vi "PH_Powermeter_BaseClass.ProcEvents.vi"(0 "i ref in":refnum<vi>, 5 "error in":errorcluster) -> (14 "i ref out":refnum<vi>, 19 "error out":errorcluster)   [LabVIEW 2014, in "PH_Powermeter_BaseClass.lvlib"]
doc: "This method is used to define the events the object will listen to. Add your own events here."
uses:
  PH_Powermeter_BaseClass.lvlib
  CSCore/BaseProcess/BaseProcess.event definition.ctl
  CSCore/CAEObj/CAEObj.event definition.ctl
  CSCore/BaseProcess/BaseProcess.descriptor string definition.ctl
  CSCore/BaseProcess/BaseProcess.lvlib
  CSCore/CAEObj/CAEObj.lvlib
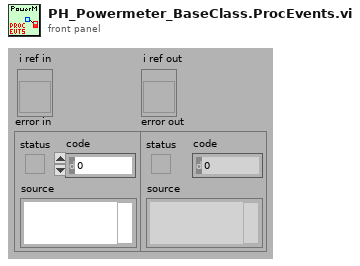
[diagram p1: front panel]
types:
  T1 = typedef "BaseProcess.lvlib/BaseProcess.event definition.ctl" = cluster{"CAEEvtDef":T2, "Data Descriptor":T3}
  T2 = typedef "CAEObj.lvlib/CAEObj.event definition.ctl" = cluster{"URL":string, "enable":bool, "ignoreResID":bool}
  T3 = typedef "BaseProcess.lvlib/BaseProcess.descriptor string definition.ctl" = string
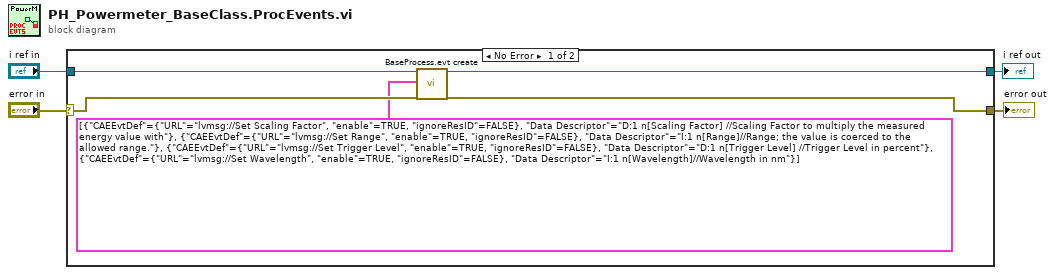
[diagram p0: block diagram]
diagram:
  n1 = case shown="No Error" "error in" {
    selector: "error in" -> [w7 w10]
    tunnel: "i ref in" -> [w6 w11]
    tunnel: [w9 w11] -> w3
    tunnel: [w8 w10] -> w2
    frame No Error {
      n2 = call "BaseProcess.evt create.vi"("i ref in"=w6, "newEvents"=T1[] [{"CAEEvtDef"={"URL"="lvmsg://Set Scaling Factor", "enable"=TRUE, "ignoreResID"=FALSE}, "Data Descriptor"="D:1 n[Scaling Factor] //Scaling Factor to multiply the measured energy value with"}, {"CAEEvtDef"={"URL"="lvmsg://Set Range", "enable"=TRUE, "ignoreResID"=FALSE}, "Data Descriptor"="I:1 n[Range]//Range; the value is coerced to the allowed range."}, {"CAEEvtDef"={"URL"="lvmsg://Set Trigger Level", "enable"=TRUE, "ignoreResID"=FALSE}, "Data Descriptor"="D:1 n[Trigger Level] //Trigger Level in percent"}, {"CAEEvtDef"={"URL"="lvmsg://Set Wavelength", "enable"=TRUE, "ignoreResID"=FALSE}, "Data Descriptor"="I:1 n[Wavelength]//Wavelength in nm"}], "error in (no error)"=w7) -> ("i ref out"=w9:refnum<vi>, "error out"=w8:errorcluster)  [unwired: 13 in, 2 out]
    }
    frame Error {
    }
  }
  "i ref out" <- w3
  "error out" <- w2
